vi "BT Example 8 - Notifier Synch.vi"() -> ()   [LabVIEW 2021]
uses:
  Support/Nodes/abs_Node/Status.ctl
  System/bt_System.lvclass
  Support/Nodes/Composites/abs_Parallel/Support/Status Calculation.ctl
  Blackboard/Blackboard.lvclass
  Support/Nodes/Decorators/Repeater/Support/Finish On - Type.ctl
  Blackboard/Blackboard.lvclass/Blackboard.ctl
  Support/Nodes/Leaves/abs_Type Leaf/abs_Type Leaf.lvclass/abs_Type Leaf.ctl
  Blackboard/Get Value Type/Get I32.vi
  <vilib>/TSA/Abstract Data Classes/Abs_Types/I32 Integer/Static Read.vi
  Blackboard/Support/Index Group.vi
  Blackboard/Support/Index Tags.vi
  Support/Nodes/Leaves/abs_Type Leaf/Properties/Write Value Class.vi
  <vilib>/TSA/Omni-Bus/Local Bus/Support/I32/Local Bus_I32.lvclass
  C:/Program Files (x86)/National Instruments/LabVIEW 2021/vi.lib/TSA/Abstract Data Classes/Abs_Types/Value/Abs_Value.lvclass
  <vilib>/TSA/Abstract Data Classes/Abs_Types/I32 Integer/Abs_I32 Integer.lvclass
  C:/Program Files (x86)/National Instruments/LabVIEW 2021/vi.lib/TSA/Abstract Data Classes/Abs_Types/Numeric/Abs_Numeric.lvclass
  Support/Nodes/Leaves/Test Boolean/Test Abs_Boolean.lvclass
  C:/Users/Tim/Documents/GitHub/LV_Behaviour_Tree/Source/Support/Nodes/abs_Node/bt_Node.lvclass
  C:/Users/Tim/Documents/GitHub/LV_Behaviour_Tree/Source/Support/Nodes/Leaves/abs_Type Leaf/abs_Type Leaf.lvclass
  <vilib>/TSA/Abstract Data Classes/Abs_Types/Boolean/Abs_Boolean.lvclass
  C:/Program Files (x86)/National Instruments/LabVIEW 2021/vi.lib/TSA/Abstract Data Classes/Abs_Types/Type/Abs_Type.lvclass
  <vilib>/TSA/Abstract Data Classes/Constants/Support/I32/I32.vi
  <vilib>/TSA/Omni-Bus/Local Bus/Support/Initialise DVR's.vi
  <vilib>/TSA/Abstract Data Classes/Functions/Math/Support/Increment/I32/Method.vi
  <vilib>/TSA/Abstract Data Classes/Functions/Compare/Support/Greater Equal/I32/Method.vi
  <vilib>/TSA/Abstract Data Classes/Abs_Types/Value/Abs_Value.lvclass
  <vilib>/TSA/Abstract Data Classes/Abs_Types/Type/Abs_Type.lvclass
  <vilib>/TSA/Omni-Bus/Local Bus/Support/DBL/Local Bus_DBL.lvclass
  <vilib>/TSA/Omni-Bus/Local Bus/Support/SGL/Local Bus_SGL.lvclass
  <vilib>/TSA/Omni-Bus/Local Bus/Support/EXT/Local Bus_EXT.lvclass
  <vilib>/TSA/Omni-Bus/Local Bus/Support/Bool/Local Bus_Boolean.lvclass
  <vilib>/TSA/Omni-Bus/Local Bus/Support/STR/Local Bus_String.lvclass
  <vilib>/TSA/Omni-Bus/Local Bus/Support/Variant/Local Bus_Variant.lvclass
  <vilib>/TSA/Omni-Bus/Local Bus/Support/WFM/Local Bus_Waveform.lvclass
  <vilib>/TSA/Omni-Bus/Local Bus/Support/Time/Local Bus_Time.lvclass
  <vilib>/TSA/Omni-Bus/Local Bus/Support/U8/Local Bus_U8.lvclass
  <vilib>/TSA/Omni-Bus/Local Bus/Support/U16/Local Bus_U16.lvclass
  <vilib>/TSA/Omni-Bus/Local Bus/Support/U32/Local Bus_U32.lvclass
  <vilib>/TSA/Omni-Bus/Local Bus/Support/U64/Local Bus_U64.lvclass
  <vilib>/TSA/Omni-Bus/Local Bus/Support/I8/Local Bus_I8.lvclass
  <vilib>/TSA/Omni-Bus/Local Bus/Support/I16/Local Bus_I16.lvclass
  <vilib>/TSA/Omni-Bus/Local Bus/Support/I64/Local Bus_I64.lvclass
  <vilib>/TSA/Omni-Bus/Local Bus/Support/CSGL/Local Bus_CSGL.lvclass
  <vilib>/TSA/Omni-Bus/Local Bus/Support/CDBL/Local Bus_CDBL.lvclass
  <vilib>/TSA/Omni-Bus/Local Bus/Support/CEXT/Local Bus_CEXT.lvclass
  <vilib>/TSA/Omni-Bus/Local Bus/Support/Type/Local Bus_Type.lvclass
  BT.lvlib
  Support/Nodes/Composites/abs_Parallel/bt_Parallel.lvclass
  Support/Nodes/Decorators/Repeater/bt_Repeater.lvclass
  C:/Program Files (x86)/National Instruments/LabVIEW 2021/vi.lib/TSA/Abstract Data Classes/Abs_Types/Integer/Abs_Integer.lvclass
  C:/Program Files (x86)/National Instruments/LabVIEW 2021/vi.lib/TSA/Abstract Data Classes/Abs_Types/I32 Integer/Abs_I32 Integer.lvclass
  <vilib>/TSA/Abstract Data Classes/Functions/Math/Support/Increment/I32/Increment_I32.lvclass
  <vilib>/TSA/Abstract Data Classes/Constants/Support/I32/Const_I32.lvclass
  <vilib>/TSA/Abstract Data Classes/Functions/Compare/Support/Greater Equal/I32/Greater Equal_I32.lvclass
  Support/Nodes/abs_Node/bt_Node.lvclass
panel:
  out "Tags Table":string[][](table)
  out "Values":u32[](array[numeric])
  out "error out":errorcluster
  in  "stop":bool
  out "Status":T1
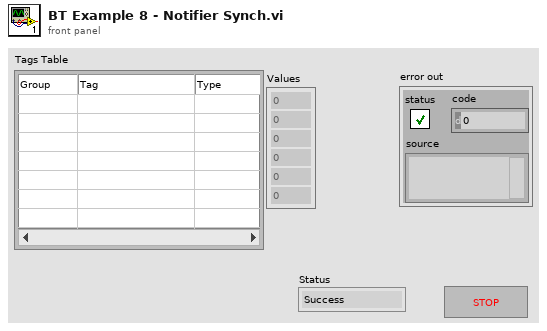
[diagram p1: front panel]
types:
  T1 = typedef "BT.lvlib/bt_Node.lvclass/Status.ctl" = enum16{"Success", "Failure", "Running"}
  T2 = typedef "BT.lvlib/bt_Repeater.lvclass/Finish On - Type.ctl" = enum16{"Success", "Failure", "Never"}
  T3 = typedef "BT.lvlib/bt_Parallel.lvclass/Status Calculation.ctl" = enum16{"Succeed on All Succeed", "Failure on All Failure", "Succeed on Any Succeed", "Failure on Any Failure"}
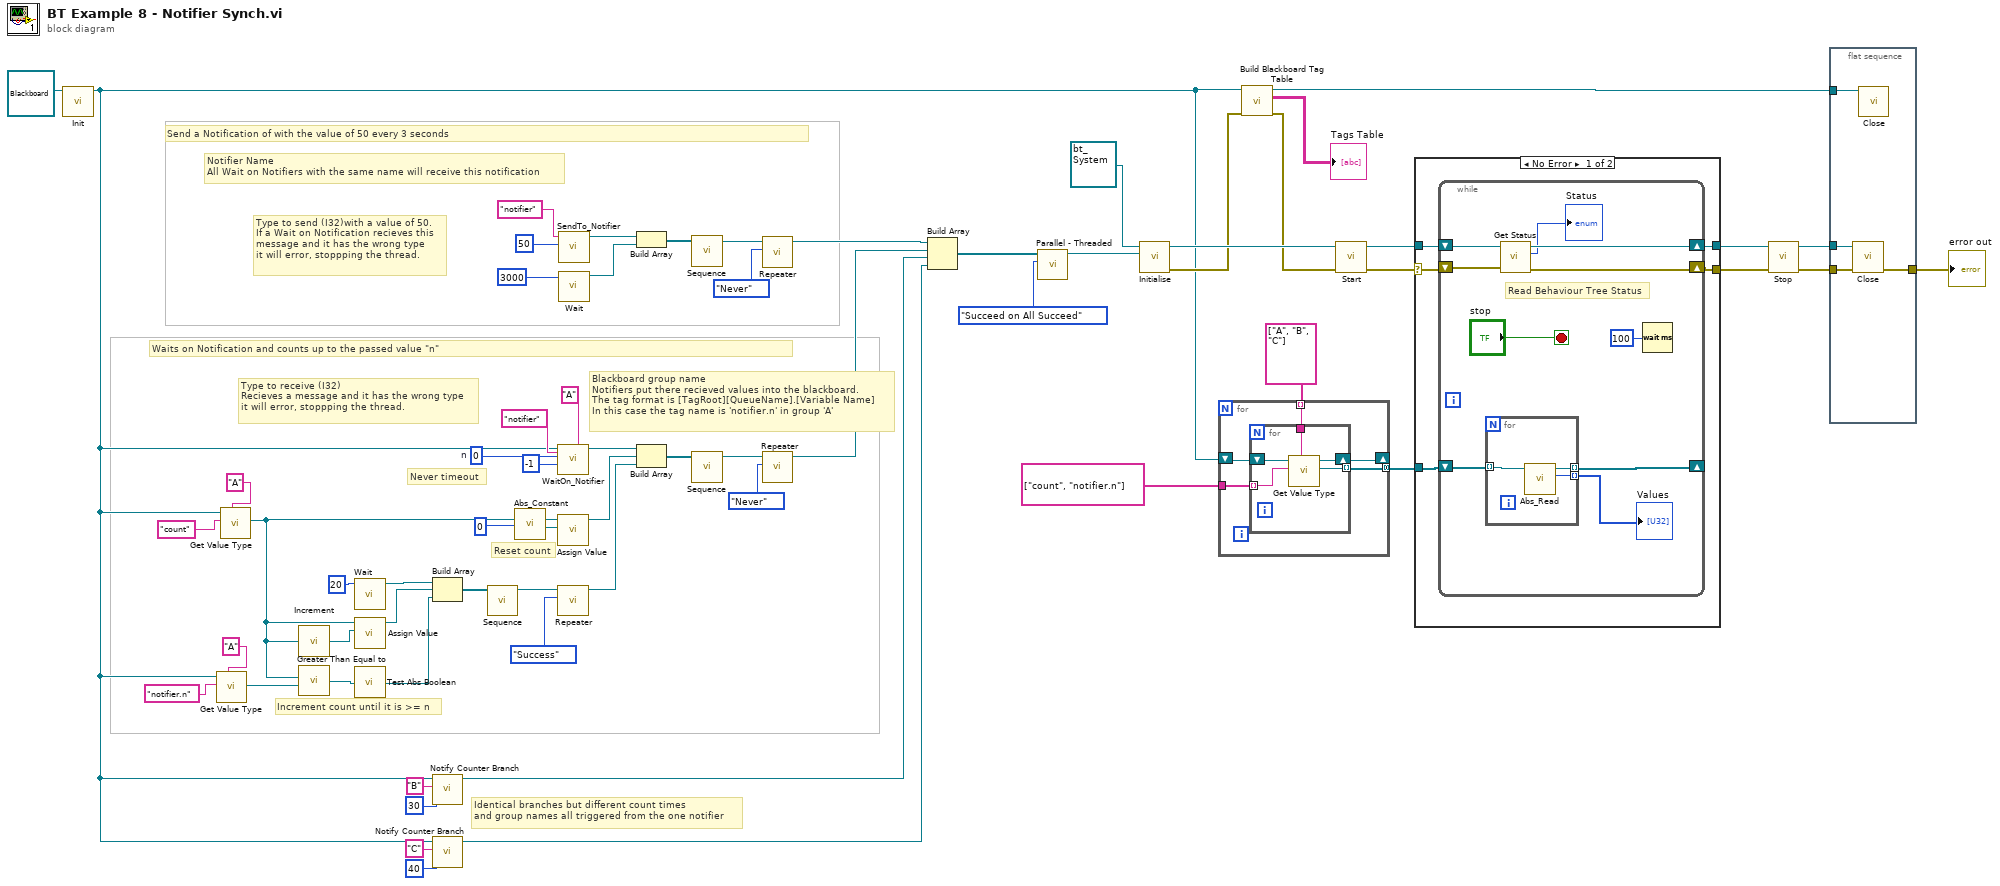
[diagram p0: block diagram]
diagram:
  w18 = 0  # n
  # "Waits on Notification and counts up to the passed value \"n\""
  # "Increment count until it is >= n"
  # "Reset count"
  # "Identical branches but different count times\nand group names all triggered from the one notifier"
  # "Blackboard group name\nNotifiers put there recieved values into the blackboard.\nThe tag format is [TagRoot][QueueName].[Variable Name]\nIn this case the tag name is 'notifier.n' in group 'A'"
  # "Never timeout"
  # "Type to receive (I32)\nRecieves a message and it has the wrong type\nit will error, stoppping the thread."
  # "Notifier Name\nAll Wait on Notifiers with the same name will receive this notification"
  # "Type to send (I32)with a value of 50.\nIf a Wait on Notification recieves this\nmessage and it has the wrong type\nit will error, stoppping the thread."
  # "Send a Notification of with the value of 50 every 3 seconds"
  n1 = call-dynamic "Init.vi"("bt_Blackboard in"=refnum<class "Blackboard.lvclass"> refnum) -> ("bt_Blackboard out"=w3:refnum<class "Blackboard.lvclass">)  [unwired: 9 in, 1 out]
  n2 = call-poly "Get Value Type.vi"("Tag Group"="A" ("Blackboard Group"), "Tag"="notifier.n", "Blackboard in"=w3) -> ("Value"=w11:refnum<class "Abs_I32 Integer.lvclass">)  [unwired: 5 in, 3 out]
  n3 = call-poly "Get Value Type.vi"("Tag Group"="A" ("Blackboard Group"), "Tag"="count", "Blackboard in"=w3) -> ("Value"=w12:refnum<class "Abs_I32 Integer.lvclass">)  [unwired: 5 in, 3 out]
  n4 = call-poly <vilib>:"Increment.vi"("Value"=w12) -> ("Result"=w35:refnum<class "Abs_I32 Integer.lvclass">)  [unwired: 4 in]
  n5 = call-poly <vilib>:"Greater Than Equal to.vi"("Value B"=w11, "Value A"=w12) -> ("Result"=w33:refnum<class "Abs_Boolean.lvclass">)  [unwired: 4 in]
  n6 = call "Wait.vi"("Time (ms)"=u32 20) -> ("Node Out"=w30:refnum<class "bt_Node.lvclass">)  [unwired: 10 in]
  n7 = call "Assign Value.vi"("Assigned Value"=w35, "Value"=w12) -> ("Node Out"=w34:refnum<class "bt_Node.lvclass">)  [unwired: 9 in]
  n8 = call "Test Abs Boolean.vi"("Abs_Boolean.lvclass"=w33) -> ("abs_Node"=w32:refnum<class "bt_Node.lvclass">)  [unwired: 4 in]
  n9 = Build Array(w30, w34, w32) -> (w40:refnum<class "bt_Node.lvclass">[])
  n10 = call "Notify Counter Branch.vi"("Time (ms)"=u32 30, "Blackboard Group"="B", "Blackboard in"=w3) -> ("bt_Node out"=w13:refnum<class "bt_Node.lvclass">)  [unwired: 8 in]
  n11 = call "Notify Counter Branch.vi"("Time (ms)"=u32 40, "Blackboard Group"="C", "Blackboard in"=w3) -> ("bt_Node out"=w2:refnum<class "bt_Node.lvclass">)  [unwired: 8 in]
  n12 = call "Sequence.vi"("Nodes"=w40) -> ("Node"=w41:refnum<class "bt_Node.lvclass">)  [unwired: 10 in]
  n13 = call-poly <vilib>:"Abs_Constant.vi"("Value"=0 ("n")) -> ("Constant"=w36:refnum<class "Abs_I32 Integer.lvclass">)  [unwired: 4 in]
  n14 = call "WaitOn_Notifier.vi"("Blackboard Group"="A", "Notifier Name"="notifier" ("Name"), "Timeout (ms)"=-1, "Message Type"=w18, "bt_Blackboard in"=w3) -> ("Node Out"=w17:refnum<class "bt_Node.lvclass">)  [unwired: 5 in, 1 out]
  n15 = call "Assign Value.vi"("Assigned Value"=w36, "Value"=w12) -> ("Node Out"=w31:refnum<class "bt_Node.lvclass">)  [unwired: 9 in]
  n16 = call "Repeater.vi"("Finish On"=Finish_On_-_Type."Success", "Node In"=w41) -> ("Node Out"=w42:refnum<class "bt_Node.lvclass">)  [unwired: 9 in]
  n17 = call "SendTo_Notifier.vi"("Message"=50, "Queue Name"="notifier" ("Name")) -> ("Node Out"=w56:refnum<class "bt_Node.lvclass">)  [unwired: 9 in]
  n18 = call "Wait.vi"("Time (ms)"=u32 3000) -> ("Node Out"=w53:refnum<class "bt_Node.lvclass">)  [unwired: 10 in]
  n19 = Build Array(w56, w53) -> (w55:refnum<class "bt_Node.lvclass">[])
  n20 = Build Array(w17, w31, w42) -> (w44:refnum<class "bt_Node.lvclass">[])
  n21 = call "Sequence.vi"("Nodes"=w55) -> ("Node"=w21:refnum<class "bt_Node.lvclass">)  [unwired: 10 in]
  n22 = call "Sequence.vi"("Nodes"=w44) -> ("Node"=w43:refnum<class "bt_Node.lvclass">)  [unwired: 10 in]
  n23 = call "Repeater.vi"("Finish On"=Finish_On_-_Type."Never", "Node In"=w21) -> ("Node Out"=w20:refnum<class "bt_Node.lvclass">)  [unwired: 9 in]
  n24 = call "Repeater.vi"("Finish On"=Finish_On_-_Type."Never", "Node In"=w43) -> ("Node Out"=w51:refnum<class "bt_Node.lvclass">)  [unwired: 9 in]
  n25 = Build Array(w20, w51, w13, w2) -> (w58:refnum<class "bt_Node.lvclass">[])
  n26 = call "Parallel - Threaded.vi"("Status Calculation"=Status_Calculation."Succeed on All Succeed", "Nodes"=w58) -> ("Node"=w57:refnum<class "bt_Node.lvclass">)  [unwired: 9 in]
  n27 = call "Initialise.vi"("Behaviour Tree"=w57, "bt_System in"=refnum<class "bt_System.lvclass"> refnum) -> ("error out"=w23:errorcluster, "bt_System out"=w26:refnum<class "bt_System.lvclass">)  [unwired: 8 in]
  n28 = for {
    shift-right: [w68] -> _
    shift-left: w3 -> [w69]
    tunnel: string[] ["A", "B", "C"] ("Blackboard Group") -> [w67] mode=indexing
    tunnel: [w66] -> w9 mode=concatenating
    tunnel: string[] ["count", "notifier.n"] ("Tag") -> [w65]
    n29 = for {
      shift-right: [w73] -> w68
      shift-left: w69 -> [w74]
      tunnel: w67 -> [w72]
      tunnel: [w71] -> w66 mode=indexing
      tunnel: w65 -> [w70] mode=indexing
      n30 = call-poly "Get Value Type.vi"("Tag Group"=w72, "Tag"=w70, "Blackboard in"=w74) -> ("Value"=w71:refnum<class "Abs_I32 Integer.lvclass">, "Blackboard out"=w73:refnum<class "Blackboard.lvclass">)  [unwired: 5 in, 2 out]
    }
  }
  n31 = call "Build Blackboard Tag Table.vi"("error in (no error)"=w23, "Blackboard in"=w3) -> ("error out"=w25:errorcluster, "Table"=→"Tags Table":string[][], "Blackboard out"=w24:refnum<class "Blackboard.lvclass">)  [unwired: 6 in, 1 out]
  n32 = call "Start.vi"("error in (no error)"=w25, "bt_System in"=w26) -> ("error out"=w47:errorcluster, "bt_System out"=w63:refnum<class "bt_System.lvclass">)  [unwired: 8 in]
  n33 = case shown="No Error" w47 {
    selector: w47 -> [w77 w93]
    tunnel: w63 -> [w79 w94]
    tunnel: [w78 w94] -> w60
    tunnel: [w76 w93] -> w45
    tunnel: w9 -> [w75 _]
    frame No Error {
      n34 = while {
        shift-right: [w87] -> w78
        shift-left: w79 -> [w88]
        shift-right: [w83] -> w76
        shift-left: w77 -> [w84]
        shift-right: [w81] -> _
        shift-left: w75 -> [w80]
        stop <- "stop" stop-if-true
        # "Read Behaviour Tree Status"
        n35 = for {
          tunnel: [w92] -> w82 mode=indexing
          tunnel: [w91] -> w81 mode=indexing
          tunnel: w80 -> [w90] mode=indexing
          n36 = call-poly <vilib>:"Abs_Read.vi"("Abs_I32 Integer in"=w90) -> ("Value"=w92:i32, "Abs_I32 Integer out"=w91:refnum<class "Abs_I32 Integer.lvclass">)  [unwired: 8 in, 1 out]
        }
        "Values" <- w82
        n37 = call "Get Status.vi"("error in (no error)"=w84, "bt_System in"=w88) -> ("error out"=w83:errorcluster, "Status"=→"Status":T1, "bt_System out"=w87:refnum<class "bt_System.lvclass">)  [unwired: 7 in]
        n38 = Wait (ms)(milliseconds to wait=u32 100) -> ()  [unwired: 1 out]
      }
    }
    frame Error {
    }
  }
  n39 = call "Stop.vi"("error in (no error)"=w45, "bt_System in"=w60) -> ("error out"=w61:errorcluster, "bt_System out"=w62:refnum<class "bt_System.lvclass">)  [unwired: 8 in]
  n40 = flat-sequence {
    tunnel: w62 -> [w98]
    tunnel: w61 -> [w97]
    tunnel: [w96] -> w46
    tunnel: w24 -> [w95]
    frame #0 {
      n41 = call-dynamic "Close.vi"("error in (no error)"=w97, "bt_System in"=w98) -> ("error out"=w96:errorcluster)  [unwired: 8 in, 1 out]
      n42 = call-dynamic "Close.vi"("bt_Blackboard in"=w95) -> ()  [unwired: 9 in, 2 out]
    }
  }
  "error out" <- w46
